vi "UI LED.vi"(8 "error in":errorcluster) -> (0 "error out":errorcluster)   [LabVIEW 2019, in "LED.lvlib"]
uses:
  LED.lvlib
  User Event/Controls/UE Abort Action.ctl
  SubVI/Image Para.ctl
  Camera/Andor/SubVI/seletion.ctl
  <vilib>/Utility/miscctls.llb/LVPointTypeDef.ctl
  SubVI/ADC Channel.ctl
  <vilib>/Utility/error.llb/Error Cluster From Error Code.vi
  <vilib>/ErrorRing/Error Ring.xnode
  Queues/Queues.lvlib
  Camera/Andor/Andor.lvlib
panel:
  in  "LED Control":T1={"LED"=enum."No Selection", "Power (%)"={"BrLED"=15, "Blue"=15, "Green"=15, "Red"=15, "UV"=15}} {"Power (%)"."UV" min=15 max=100; "Power (%)"."Red" min=15 max=100; "Power (%)"."Green" min=15 max=100; "Power (%)"."Blue" min=15 max=100; "Power (%)"."BrLED" min=15 max=100}
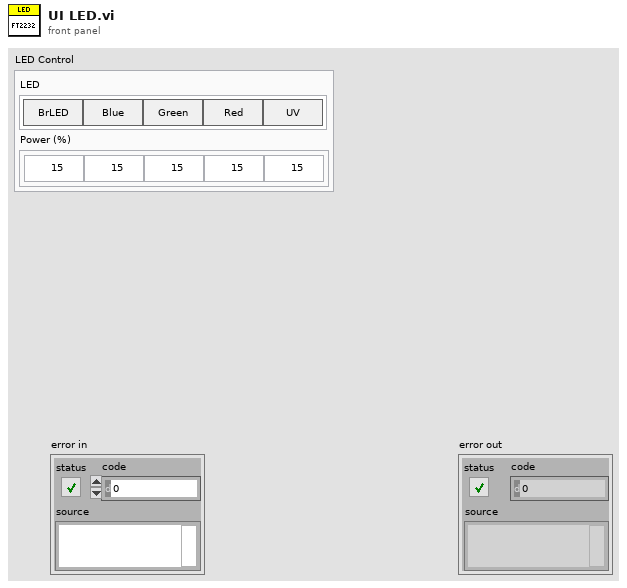
[diagram p1: front panel]
types:
  T1 = cluster{"LED":enum32{"No Selection", "BrLED", "Blue", "Green", "Red", "UV"}, "Power (%)":cluster{"BrLED":u8, "Blue":u8, "Green":u8, "Red":u8, "UV":u8}}
  T2 = cluster{"Initialize Sucess?":bool, "LED Control":cluster{"LED color":enum32{"BrLED", "Blue", "Green", "Red", "UV"}, "LED Power":u8}}
  T3 = typedef "UE Abort Action.ctl" = enum16{"Create", "Get", "Destroy"}
  T4 = typedef "LED.lvlib/Image Para.ctl" = cluster{"Marker":T5, "Power(Amp)":u8, "set shutter(s)":dbl, "Cube":enum16{"1", "2", "3", "4", "5", "6", "7", "8"}}
  T5 = typedef "Andor.lvlib/seletion.ctl" = enum16{"None", "Red", "Green", "Blue", "UV", "Green Laser", "Blue-Red", "UV-Red", "BF", "UV-IR"}
  T6 = cluster{"LED color":enum32{"BrLED", "Blue", "Green", "Red", "UV"}, "LED Power":u8}
  T7 = enum32{"No Selection", "BrLED", "Blue", "Green", "Red", "UV"}
  T8 = typedef "LVPointTypeDef.ctl" = cluster{"Horizontal":i16, "Vertical":i16}
  T9 = enum16{"LED Initial", "LED On", "LED Off", "LED Change", "LED Close", "ADC Read"}
  T10 = cluster{"return":i32, "numDev":u32, "ftHandleFluChA":u32, "ftHandleFluChB":u32, "ftHandleBriChA":u32, "ftHandleBriChB":u32, "ftHandelADCChA":u32, "ftHandleADCChB":u32}
  T11 = typedef "LED.lvlib/SEQ Data.ctl" = cluster{"Initialize Sucess?":bool, "BL2 Regulator":dbl, "BL1 Regulator":dbl, "Blood Sensor 1":dbl, "Blood Sensor 2":dbl, "Air Pressure Sensor":dbl, "Force Snesor 1":u32, "Force Snesor 2":u32, "VI Refnum":refnum<vi>}
  T12 = typedef "Rendezvous RefNum" = refnum<k1>
  T13 = typedef "LED.lvlib/ADC Channel.ctl" = enum16{"BL2 Regulator", "BL1 Regulator", "Blood Sensor 1", "Blood Sensor 2", "Air Pressure Sensor", "Force Sensor 1", "Force Snesor 2"}
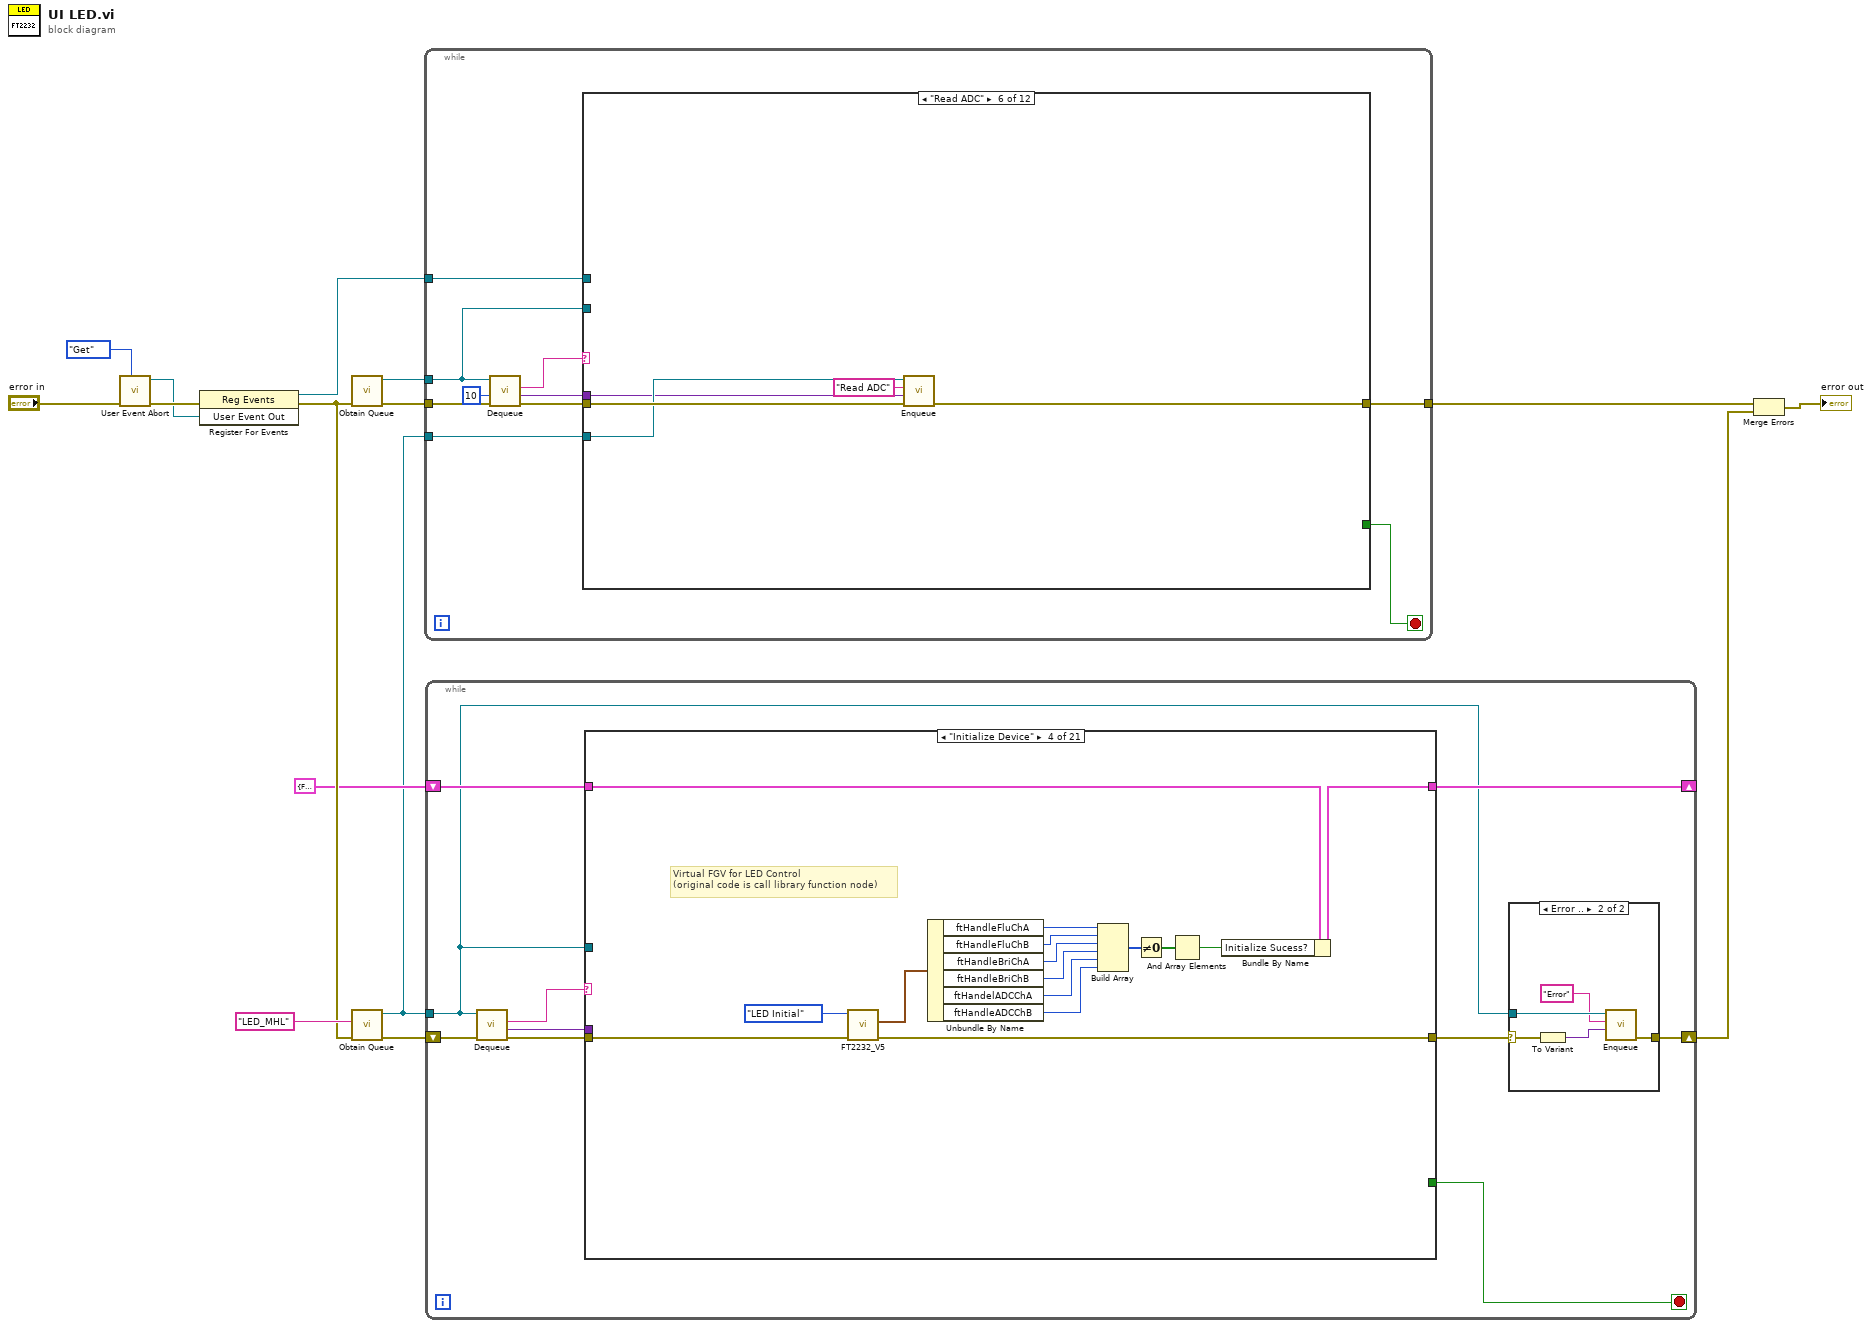
[diagram p0: block diagram]
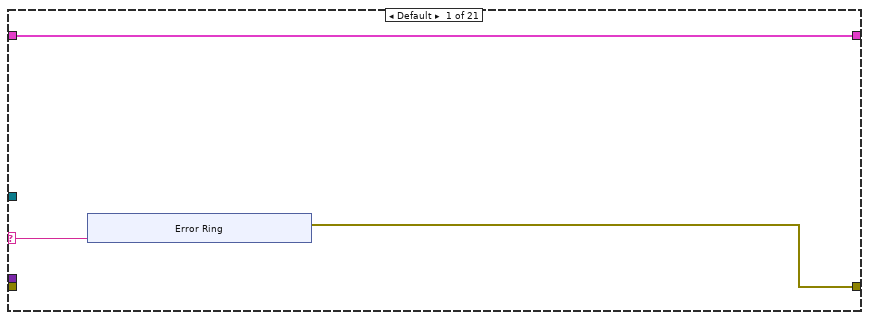
[diagram p2: hidden frame]
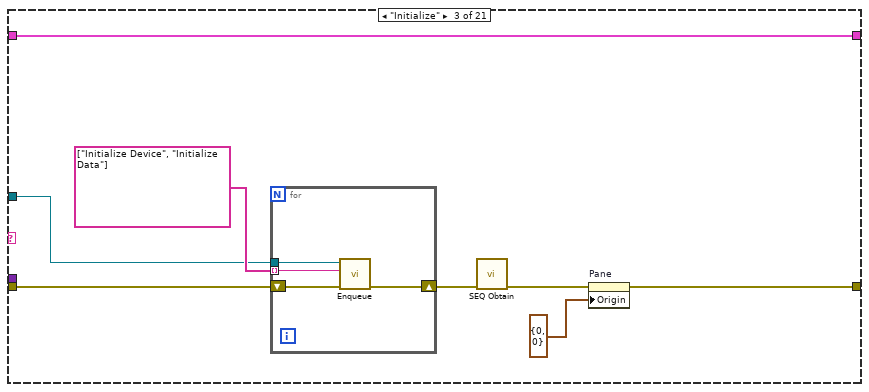
[diagram p4: hidden frame]
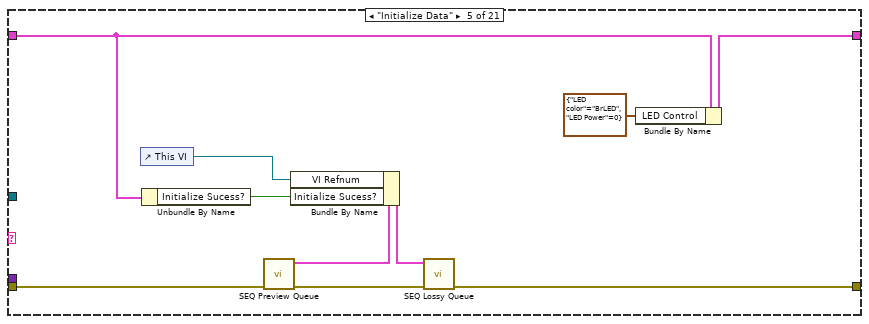
[diagram p5: hidden frame]
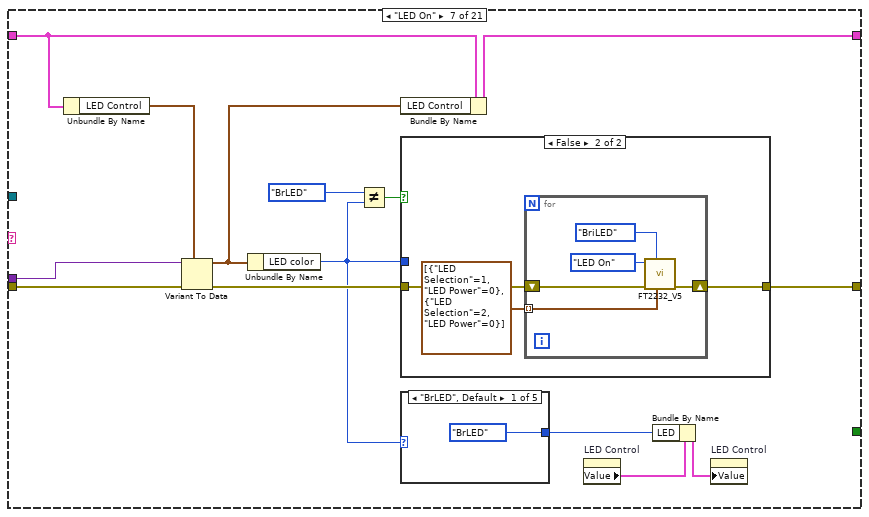
[diagram p7: hidden frame]
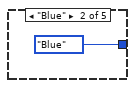
[diagram p8: hidden frame]
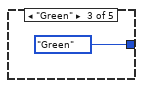
[diagram p9: hidden frame]
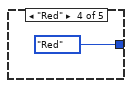
[diagram p10: hidden frame]
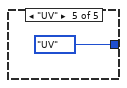
[diagram p11: hidden frame]
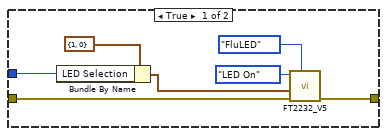
[diagram p12: hidden frame]
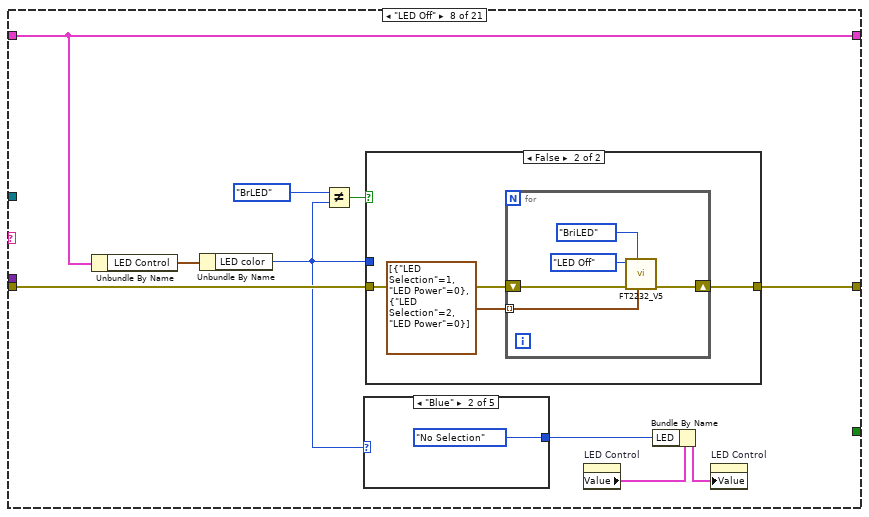
[diagram p13: hidden frame]
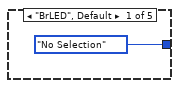
[diagram p14: hidden frame]
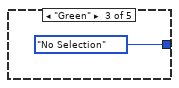
[diagram p15: hidden frame]
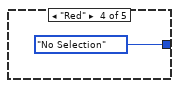
[diagram p16: hidden frame]
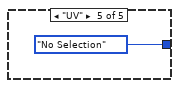
[diagram p17: hidden frame]
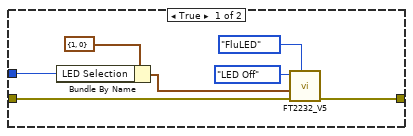
[diagram p18: hidden frame]
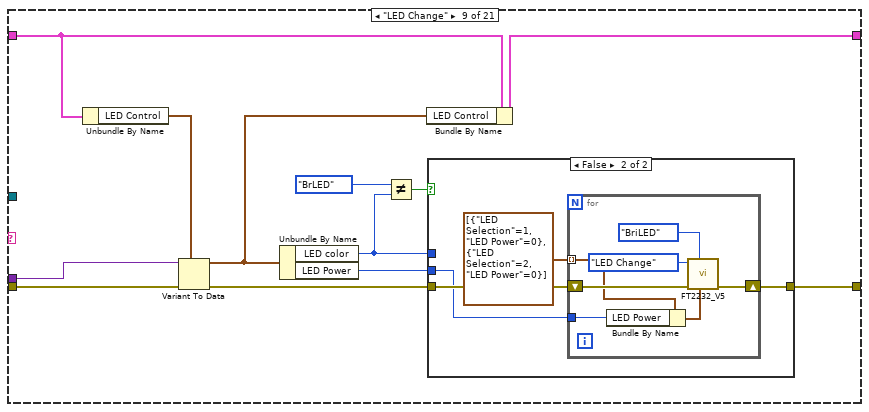
[diagram p19: hidden frame]
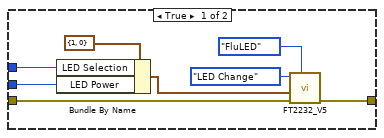
[diagram p20: hidden frame]
diagram:
  n1 = call "User Event Abort.vi"("Action"=UE_Abort_Action."Get", "Error In"="error in") -> ("Error Out"=w13:errorcluster, "User Event Out"=w12:refnum<user-event>)  [unwired: 8 in]
  n2 = register-events(error in=w13, w12) -> (reference out=w11:refnum<event-registration>, error out=w6:errorcluster)  [unwired: 1 in]
  n3 = call "Obtain Queue.vi"("Error In"=w6) -> ("Error Out"=w10:errorcluster, "Queue out"=w9:refnum<queue>)  [unwired: 9 in]
  n4 = call "Obtain Queue.vi"("Error In"=w6, "Queue Name"="LED_MHL") -> ("Error Out"=w7:errorcluster, "queue out"=w1:refnum<queue>)  [unwired: 8 in]
  n5 = while {
    tunnel: w10 -> [w25]
    tunnel: w9 -> [w20]
    tunnel: [w19] -> w5
    tunnel: w11 -> [w18]
    tunnel: w1 -> [w16]
    stop <- w17 stop-if-true
    n6 = call "Dequeue.vi"("Error In"=w25, "timeout in ms (-1)"=10, "Queue in"=w20) -> ("Error Out"=w24:errorcluster, "Data"=w22:variant, "State"=w23:string)  [unwired: 5 in, 1 out]
    n7 = case shown="\"Read ADC\"" w23 {
      selector: w23 -> [w26 _ _ _ _ _ _ _ _ _ _ _]
      tunnel: w24 -> [w29 w33 w52 w71 w77 w89 w93 w97 w100 w104 w108 w116]
      tunnel: w22 -> [_ _ w50 w69 _ w87 _ _ _ _ _ _]
      tunnel: w20 -> [_ _ _ _ _ _ _ _ _ _ _ _]
      tunnel: [w29 w32 w47 w66 w80 w86 w92 w96 w98 w103 w107 w115] -> w19
      tunnel: w18 -> [_ _ _ _ _ _ _ _ _ _ _ w114]
      tunnel: [_ _ _ _ _ _ _ _ _ _ TRUE _] -> w17
      tunnel: w16 -> [_ w31 w46 w65 w79 w88 w91 w95 w99 w102 w106 _]
      frame "Typo", Default {
        n8 = Concatenate Strings("Typo: " ("string"), w26) -> (w28:string)
        n9 = One Button Dialog(message=w28) -> ()  [unwired: 1 in, 1 out]
      }
      frame "Initialize" {
        n10 = for {
          tunnel: w31 -> [w35]
          shift-right: [w36] -> w32
          shift-left: w33 -> [w37]
          tunnel: string[] ["Initialize"] -> [w34] mode=indexing
          n11 = call "Enqueue.vi"("Error In"=w37, "State"=w34, "Queue in"=w35) -> ("Error Out"=w36:errorcluster)  [unwired: 7 in, 1 out]
        }
      }
      frame "LED On" {
        w44 = variant ("element")
        n12 = Variant To Data(error in=w52, type=T4 {"Marker"=enum."None", "Power(Amp)"=0, "set shutter(s)"=0.001, "Cube"=enum."2"} ("Color&Power control"), Variant=w50) -> (data=w48:T4, error out=w49:errorcluster)
        n13 = call "Image Para Extract.vi"("error in"=w49, "Image Para"=w48) -> ("error out"=w41:errorcluster, "LED Control out"=w39:T6)  [unwired: 6 in, 2 out]
        n14 = call "Power Convert.vi"("error in"=w41, "LED Control in"=w39) -> ("error out"=w40:errorcluster, "LED Control out"=w38:T6)  [unwired: 8 in]
        n15 = To Variant(anything=w38) -> (Variant=w45:variant)
        n16 = Build Array(w44, w44, w45, w45) -> (w43:variant[])
        n17 = for {
          tunnel: w46 -> [w55]
          shift-right: [w56] -> w47
          shift-left: w40 -> [w57]
          tunnel: w43 -> [w54] mode=indexing
          tunnel: string[] ["LED Zero", "LED Off", "LED Change", "LED On"] -> [w53] mode=indexing
          n18 = call "Enqueue.vi"("Error In"=w57, "Data"=w54, "State"=w53, "Queue in"=w55) -> ("Error Out"=w56:errorcluster)  [unwired: 6 in, 1 out]
        }
      }
      frame "LED Change" {
        n19 = Variant To Data(error in=w71, type=T4 {"Marker"=enum."None", "Power(Amp)"=0, "set shutter(s)"=0.001, "Cube"=enum."2"} ("Color&Power control"), Variant=w69) -> (data=w67:T4, error out=w68:errorcluster)
        n20 = call "Image Para Extract.vi"("error in"=w68, "Image Para"=w67) -> ("error out"=w61:errorcluster, "LED Control out"=w59:T6)  [unwired: 6 in, 2 out]
        n21 = call "Power Convert.vi"("error in"=w61, "LED Control in"=w59) -> ("error out"=w60:errorcluster, "LED Control out"=w58:T6)  [unwired: 8 in]
        n22 = To Variant(anything=w58) -> (Variant=w62:variant)
        n23 = Build Array(w62) -> (w64:variant[])
        n24 = for {
          tunnel: w65 -> [w74]
          shift-right: [w75] -> w66
          shift-left: w60 -> [w76]
          tunnel: w64 -> [w73] mode=indexing
          tunnel: string[] ["LED Change"] -> [w72] mode=indexing
          n25 = call "Enqueue.vi"("Error In"=w76, "Data"=w73, "State"=w72, "Queue in"=w74) -> ("Error Out"=w75:errorcluster)  [unwired: 6 in, 1 out]
        }
      }
      frame "LED Off" {
        n26 = for {
          tunnel: w79 -> [w82]
          shift-right: [w83] -> w80
          shift-left: w77 -> [w84]
          tunnel: string[] ["LED Zero", "LED Off"] -> [w81] mode=indexing
          n27 = call "Enqueue.vi"("Error In"=w84, "State"=w81, "Queue in"=w82) -> ("Error Out"=w83:errorcluster)  [unwired: 7 in, 1 out]
        }
      }
      frame "Read ADC" {
        n28 = call "Enqueue.vi"("Error In"=w89, "Data"=w87, "State"="Read ADC", "Queue in"=w88) -> ("Error Out"=w86:errorcluster)  [unwired: 6 in, 1 out]
      }
      frame "Read BL2 Regulator" {
        n29 = call "Enqueue.vi"("Error In"=w93, "State"="Read BL2 Regulator", "Queue in"=w91) -> ("Error Out"=w92:errorcluster)  [unwired: 7 in, 1 out]
      }
      frame "Read Force Sensor" {
        n30 = call "Enqueue.vi"("Error In"=w97, "State"="Read Force Sensor 1", "Queue in"=w95) -> ("Error Out"=w96:errorcluster)  [unwired: 7 in, 1 out]
      }
      frame "Stop Read" {
        n31 = Flush Queue(queue=w99, error in (no error)=w100) -> (error out=w98:errorcluster)  [unwired: 2 out]
      }
      frame "Rendezvous Acquire" {
        n32 = call "Enqueue.vi"("Error In"=w104, "State"="Rendezvous Acquire", "Queue in"=w102) -> ("Error Out"=w103:errorcluster)  [unwired: 7 in, 1 out]
      }
      frame "Close" {
        n33 = for {
          tunnel: w106 -> [w111]
          shift-right: [w112] -> w107
          shift-left: w108 -> [w113]
          tunnel: string[] ["LED Zero", "LED Off", "Close"] -> [w110] mode=indexing
          n34 = call "Enqueue.vi"("Error In"=w113, "State"=w110, "Queue in"=w111) -> ("Error Out"=w112:errorcluster)  [unwired: 7 in, 1 out]
        }
      }
      frame "Idle" {
        n35 = event shown="[1] \"LED Control.LED\": Value Change" {
          selector: w114 -> [_ _ w163]
          dyn-events: _ -> [_ _ _]
          timeout: 10 -> [_ _ _]
          tunnel: w116 -> [w118 w121 w161]
          tunnel: [w118 w120 w162] -> w115
          event Timeout {
            n36 = event-data() -> ()  [unwired: 1 in, 3 out]
          }
          event "LED Control.LED": Value Change {
            n37 = event-data() -> ("NewVal"=w122:T7)  [unwired: 1 in, 5 out]
            n38 = case shown="\"No Selection\", Default" w122 {
              tunnel: w121 -> [w124 w131 w134 w141 w148 w155]
              tunnel: [w123 w130 w133 w140 w147 w154] -> w120
              tunnel: "LED Control" -> [_ w129 w132 w139 w146 w153]
              frame "No Selection", Default {
                n39 = call "LED Off.vi"("Error In"=w124) -> ("Error Out"=w123:errorcluster)  [unwired: 10 in]
              }
              frame "BrLED" {
                n40 = Unbundle By Name(w129) -> ("Power (%).BrLED"=w127:u8)
                n41 = Bundle By Name(cluster=T4 {"Marker"=enum."None", "Power(Amp)"=15, "set shutter(s)"=0.001, "Cube"=enum."1"} ("Image Para"), "Marker"=seletion."BF", "Power(Amp)"=w127) -> (w125:T4)
                n42 = call "LED On.vi"("Error In"=w131, "Image Para"=w125) -> ("Error Out"=w130:errorcluster)  [unwired: 9 in]
              }
              frame "Blue" {
                n43 = Unbundle By Name(w132) -> ("Power (%).Blue"=w137:u8)
                n44 = Bundle By Name(cluster=T4 {"Marker"=enum."None", "Power(Amp)"=15, "set shutter(s)"=0.001, "Cube"=enum."1"} ("Image Para"), "Marker"=seletion."Blue", "Power(Amp)"=w137) -> (w135:T4)
                n45 = call "LED On.vi"("Error In"=w134, "Image Para"=w135) -> ("Error Out"=w133:errorcluster)  [unwired: 9 in]
              }
              frame "Green" {
                n46 = Unbundle By Name(w139) -> ("Power (%).Green"=w144:u8)
                n47 = Bundle By Name(cluster=T4 {"Marker"=enum."None", "Power(Amp)"=15, "set shutter(s)"=0.001, "Cube"=enum."1"} ("Image Para"), "Marker"=seletion."Green", "Power(Amp)"=w144) -> (w142:T4)
                n48 = call "LED On.vi"("Error In"=w141, "Image Para"=w142) -> ("Error Out"=w140:errorcluster)  [unwired: 9 in]
              }
              frame "Red" {
                n49 = Unbundle By Name(w146) -> ("Power (%).Red"=w151:u8)
                n50 = Bundle By Name(cluster=T4 {"Marker"=enum."None", "Power(Amp)"=15, "set shutter(s)"=0.001, "Cube"=enum."1"} ("Image Para"), "Marker"=seletion."Red", "Power(Amp)"=w151) -> (w149:T4)
                n51 = call "LED On.vi"("Error In"=w148, "Image Para"=w149) -> ("Error Out"=w147:errorcluster)  [unwired: 9 in]
              }
              frame "UV" {
                n52 = Unbundle By Name(w153) -> ("Power (%).UV"=w158:u8)
                n53 = Bundle By Name(cluster=T4 {"Marker"=enum."None", "Power(Amp)"=15, "set shutter(s)"=0.001, "Cube"=enum."1"} ("Image Para"), "Marker"=seletion."UV", "Power(Amp)"=w158) -> (w156:T4)
                n54 = call "LED On.vi"("Error In"=w155, "Image Para"=w156) -> ("Error Out"=w154:errorcluster)  [unwired: 9 in]
              }
            }
          }
          event User Event {
            n55 = event-data() -> ()  [unwired: 1 in, 4 out]
            n56 = call "Close.vi"("Error In"=w161) -> ("Error Out"=w160:errorcluster)  [unwired: 10 in]
            n57 = Unregister For Events(event registration refnum=w163, error in=w160) -> (error out=w162:errorcluster)
          }
        }
      }
    }
  }
  n58 = while {
    tunnel: w1 -> [w165]
    shift-right: [w168] -> _
    shift-left: T2 {"Initialize Sucess?"=FALSE, "LED Control"={"LED color"=enum."BrLED", "LED Power"=0}} -> [w169]
    shift-right: [w167] -> w3
    shift-left: w7 -> [w173]
    stop <- w164 stop-if-true
    n59 = call "Dequeue.vi"("Error In"=w173, "Queue in"=w165) -> ("Error Out"=w170:errorcluster, "Data"=w171:variant, "State"=w172:string)  [unwired: 6 in, 1 out]
    n60 = case shown="\"Initialize Device\"" w172 {
      selector: w172 -> [w175 _ _ _ _ _ _ _ _ _ _ _ _ _ _ _ _ _ _ _ _]
      tunnel: w165 -> [_ _ w191 _ _ _ _ _ _ _ _ _ w406 w420 w436 _ _ _ w460 _ w471]
      tunnel: w171 -> [_ _ _ _ _ _ w233 _ w295 _ _ w375 _ _ _ _ w452 _ _ _ _]
      tunnel: w170 -> [_ w184 w192 w202 w219 w224 w235 w266 w297 w324 w355 w376 w408 w422 w438 w449 w453 w457 w461 w469 w474]
      tunnel: w169 -> [w176 w185 w189 w200 w217 w223 w232 w264 w294 w323 w356 w378 w418 w432 w447 w448 w450 w456 w458 w467 w476]
      tunnel: [w176 w185 w189 w199 w215 w223 w230 w264 w292 w323 w356 w378 w418 w432 w447 w448 w450 w456 w458 w467 w476] -> w168
      tunnel: [w174 w184 w186 w201 w218 w224 w236 w265 w298 w325 w347 w368 w413 w427 w442 w449 errorcluster {"status"=FALSE, "code"=0, "source"=""} ("Error Out") w457 w459 w468 w472] -> w166
      tunnel: [_ _ _ _ _ _ _ _ _ _ _ _ _ _ _ _ _ _ _ _ TRUE] -> w164
      frame Default {
        n61 = xnode "Error Ring"("parameter 0"=w175) -> ("error out"=w174:errorcluster)
      }
      frame "------Initialize------" {
      }
      frame "Initialize" {
        n62 = for {
          tunnel: w191 -> [w195]
          shift-right: [w196] -> w190
          shift-left: w192 -> [w197]
          tunnel: string[] ["Initialize Device", "Initialize Data"] -> [w194] mode=indexing
          n63 = call "Enqueue.vi"("Error In"=w197, "State"=w194, "Queue in"=w195) -> ("Error Out"=w196:errorcluster)  [unwired: 7 in, 1 out]
        }
        n64 = call "SEQ Obtain.vi"("error in"=w190) -> ("error out"=w188:errorcluster)  [unwired: 9 in, 1 out]
        n65 = property on="Pane" class="Pane"(error in=w188, "Origin"=T8 {"Horizontal"=0, "Vertical"=0}) -> (error out=w186:errorcluster)  [unwired: 1 in, 1 out]
      }
      frame "Initialize Device" {
        # "Virtual FGV for LED Control\n(original code is call library function node)"
        n66 = call "FT2232_V5.vi"("error in"=w202, "LED event"=T9."LED Initial") -> ("error out"=w201:errorcluster, "Initialize"=w204:T10)  [unwired: 6 in, 2 out]
        n67 = Unbundle By Name(w204) -> ("ftHandleFluChA"=w205:u32, "ftHandleFluChB"=w206:u32, "ftHandleBriChA"=w207:u32, "ftHandleBriChB"=w208:u32, "ftHandelADCChA"=w209:u32, "ftHandleADCChB"=w210:u32)
        n68 = Build Array(w205, w206, w207, w208, w209, w210) -> (w211:u32[])
        n69 = Not Equal To 0?(x=w211) -> (x != 0?=w212:bool[])
        n70 = And Array Elements(Boolean array=w212) -> (logical AND=w198:bool)
        n71 = Bundle By Name(cluster=w200, "Initialize Sucess?"=w198) -> (w199:T2)
      }
      frame "Initialize Data" {
        n72 = control-ref of="This VI"() -> (w213:refnum<vi>)
        n73 = Unbundle By Name(w217) -> ("Initialize Sucess?"=w216:bool)
        n74 = call "SEQ Preview Queue.vi"("error in"=w219) -> ("error out"=w220:errorcluster, "SEQ Data"=w221:T11)  [unwired: 9 in]
        n75 = Bundle By Name(cluster=w221, "VI Refnum"=w213, "Initialize Sucess?"=w216) -> (w222:T11)
        n76 = call "SEQ Lossy Queue.vi"("error in"=w220, "SEQ Data"=w222) -> ("error out"=w218:errorcluster)  [unwired: 9 in]
        n77 = Bundle By Name(cluster=w217, "LED Control"=T6 {"LED color"=enum."BrLED", "LED Power"=0}) -> (w215:T2)
      }
      frame "------Functions------" {
      }
      frame "LED On" {
        n78 = Unbundle By Name(w232) -> ("LED Control"=w231:T6)
        n79 = Variant To Data(error in=w235, type=w231, Variant=w233) -> (data=w229:T6, error out=w234:errorcluster)
        n80 = Unbundle By Name(w229) -> ("LED color"=w226:enum32{"BrLED", "Blue", "Green", "Red", "UV"})
        n81 = Not Equal?(x=enum32{"BrLED", "Blue", "Green", "Red", "UV"}."BrLED", y=w226) -> (x != y?=w238:bool)
        n82 = Bundle By Name(cluster=w232, "LED Control"=w229) -> (w230:T2)
        n83 = case shown="False" w238 {
          tunnel: w234 -> [w250 w253]
          tunnel: [w244 w251] -> w236
          tunnel: w226 -> [w246 _]
          frame True {
            n84 = Bundle By Name(cluster=cluster{"LED Selection":u16, "LED Power":u8} {"LED Selection"=1, "LED Power"=0} ("FulLED set"), "LED Selection"=w246) -> (w245:cluster{"LED Selection":u16, "LED Power":u8})
            n85 = call "FT2232_V5.vi"("LED selection"=enum16{"FluLED", "BriLED", "ADCDAC"}."FluLED", "error in"=w250, "FulLED set"=w245, "LED event"=T9."LED On") -> ("error out"=w244:errorcluster)  [unwired: 4 in, 3 out]
          }
          frame False {
            n86 = for {
              shift-right: [w254] -> w251
              shift-left: w253 -> [w258]
              tunnel: cluster{"LED Selection":u16, "LED Power":u8}[] [{"LED Selection"=1, "LED Power"=0}, {"LED Selection"=2, "LED Power"=0}] -> [w255] mode=indexing
              n87 = call "FT2232_V5.vi"("BriLED set"=w255, "LED selection"=enum16{"FluLED", "BriLED", "ADCDAC"}."BriLED", "error in"=w258, "LED event"=T9."LED On") -> ("error out"=w254:errorcluster)  [unwired: 4 in, 3 out]
            }
          }
        }
        n88 = case shown="\"BrLED\", Default" w226 {
          tunnel: [T7."BrLED" ("LED") T7."Blue" ("LED") T7."Green" ("LED") T7."Red" ("LED") T7."UV" ("LED")] -> w225
          frame "BrLED", Default {
          }
          frame "Blue" {
          }
          frame "Green" {
          }
          frame "Red" {
          }
          frame "UV" {
          }
        }
        n89 = property on="LED Control" class="Clust (strict)"() -> ("Value"=w228:T1)  [unwired: 2 in, 2 out]
        n90 = Bundle By Name(cluster=w228, "LED"=w225) -> (w227:T1)
        n91 = property on="LED Control" class="Clust (strict)"("Value"=w227) -> ()  [unwired: 2 in, 2 out]
      }
      frame "LED Off" {
        n92 = Unbundle By Name(w264) -> ("LED Control"=w263:T6)
        n93 = Unbundle By Name(w263) -> ("LED color"=w259:enum32{"BrLED", "Blue", "Green", "Red", "UV"})
        n94 = Not Equal?(x=enum32{"BrLED", "Blue", "Green", "Red", "UV"}."BrLED", y=w259) -> (x != y?=w268:bool)
        n95 = case shown="\"Blue\"" w259 {
          tunnel: [T7."No Selection" ("LED") T7."No Selection" ("LED") T7."No Selection" ("LED") T7."No Selection" ("LED") T7."No Selection" ("LED")] -> w260
          frame "BrLED", Default {
          }
          frame "Blue" {
          }
          frame "Green" {
          }
          frame "Red" {
          }
          frame "UV" {
          }
        }
        n96 = case shown="False" w268 {
          tunnel: w266 -> [w280 w283]
          tunnel: [w274 w282] -> w265
          tunnel: w259 -> [w276 _]
          frame True {
            n97 = Bundle By Name(cluster=cluster{"LED Selection":u16, "LED Power":u8} {"LED Selection"=1, "LED Power"=0} ("FulLED set"), "LED Selection"=w276) -> (w275:cluster{"LED Selection":u16, "LED Power":u8})
            n98 = call "FT2232_V5.vi"("LED selection"=enum16{"FluLED", "BriLED", "ADCDAC"}."FluLED", "error in"=w280, "FulLED set"=w275, "LED event"=T9."LED Off") -> ("error out"=w274:errorcluster)  [unwired: 4 in, 3 out]
          }
          frame False {
            n99 = for {
              shift-right: [w284] -> w282
              shift-left: w283 -> [w288]
              tunnel: cluster{"LED Selection":u16, "LED Power":u8}[] [{"LED Selection"=1, "LED Power"=0}, {"LED Selection"=2, "LED Power"=0}] -> [w285] mode=indexing
              n100 = call "FT2232_V5.vi"("BriLED set"=w285, "LED selection"=enum16{"FluLED", "BriLED", "ADCDAC"}."BriLED", "error in"=w288, "LED event"=T9."LED Off") -> ("error out"=w284:errorcluster)  [unwired: 4 in, 3 out]
            }
          }
        }
        n101 = property on="LED Control" class="Clust (strict)"() -> ("Value"=w262:T1)  [unwired: 2 in, 2 out]
        n102 = Bundle By Name(cluster=w262, "LED"=w260) -> (w261:T1)
        n103 = property on="LED Control" class="Clust (strict)"("Value"=w261) -> ()  [unwired: 2 in, 2 out]
      }
      frame "LED Change" {
        n104 = Unbundle By Name(w294) -> ("LED Control"=w293:T6)
        n105 = Variant To Data(error in=w297, type=w293, Variant=w295) -> (data=w291:T6, error out=w296:errorcluster)
        n106 = Unbundle By Name(w291) -> ("LED color"=w290:enum32{"BrLED", "Blue", "Green", "Red", "UV"}, "LED Power"=w289:u8)
        n107 = Not Equal?(x=enum32{"BrLED", "Blue", "Green", "Red", "UV"}."BrLED", y=w290) -> (x != y?=w300:bool)
        n108 = Bundle By Name(cluster=w294, "LED Control"=w291) -> (w292:T2)
        n109 = case shown="False" w300 {
          tunnel: w296 -> [w308 w312]
          tunnel: [w301 w311] -> w298
          tunnel: w290 -> [w304 _]
          tunnel: w289 -> [w302 w309]
          frame True {
            n110 = Bundle By Name(cluster=cluster{"LED Selection":u16, "LED Power":u8} {"LED Selection"=1, "LED Power"=0} ("FulLED set"), "LED Selection"=w304, "LED Power"=w302) -> (w303:cluster{"LED Selection":u16, "LED Power":u8})
            n111 = call "FT2232_V5.vi"("LED selection"=enum16{"FluLED", "BriLED", "ADCDAC"}."FluLED", "error in"=w308, "FulLED set"=w303, "LED event"=T9."LED Change") -> ("error out"=w301:errorcluster)  [unwired: 4 in, 3 out]
          }
          frame False {
            n112 = for {
              shift-right: [w313] -> w311
              shift-left: w312 -> [w319]
              tunnel: cluster{"LED Selection":u16, "LED Power":u8}[] [{"LED Selection"=1, "LED Power"=0}, {"LED Selection"=2, "LED Power"=0}] -> [w316] mode=indexing
              tunnel: w309 -> [w314]
              n113 = Bundle By Name(cluster=w316, "LED Power"=w314) -> (w315:cluster{"LED Selection":u16, "LED Power":u8})
              n114 = call "FT2232_V5.vi"("BriLED set"=w315, "LED selection"=enum16{"FluLED", "BriLED", "ADCDAC"}."BriLED", "error in"=w319, "LED event"=T9."LED Change") -> ("error out"=w313:errorcluster)  [unwired: 4 in, 3 out]
            }
          }
        }
      }
      frame "LED Zero" {
        n115 = Unbundle By Name(w323) -> ("LED Control"=w322:T6)
        n116 = Unbundle By Name(w322) -> ("LED color"=w321:enum32{"BrLED", "Blue", "Green", "Red", "UV"})
        n117 = Not Equal?(x=enum32{"BrLED", "Blue", "Green", "Red", "UV"}."BrLED", y=w321) -> (x != y?=w327:bool)
        n118 = case shown="True" w327 {
          tunnel: w324 -> [w335 w339]
          tunnel: [w328 w338] -> w325
          tunnel: w321 -> [w331 _]
          tunnel: u8 0 ("LED Power") -> [w329 w336]
          frame True {
            n119 = Bundle By Name(cluster=cluster{"LED Selection":u16, "LED Power":u8} {"LED Selection"=1, "LED Power"=0} ("FulLED set"), "LED Selection"=w331, "LED Power"=w329) -> (w330:cluster{"LED Selection":u16, "LED Power":u8})
            n120 = call "FT2232_V5.vi"("LED selection"=enum16{"FluLED", "BriLED", "ADCDAC"}."FluLED", "error in"=w335, "FulLED set"=w330, "LED event"=T9."LED Change") -> ("error out"=w328:errorcluster)  [unwired: 4 in, 3 out]
          }
          frame False {
            n121 = for {
              shift-right: [w340] -> w338
              shift-left: w339 -> [w346]
              tunnel: cluster{"LED Selection":u16, "LED Power":u8}[] [{"LED Selection"=1, "LED Power"=0}, {"LED Selection"=2, "LED Power"=0}] -> [w343] mode=indexing
              tunnel: w336 -> [w341]
              n122 = Bundle By Name(cluster=w343, "LED Power"=w341) -> (w342:cluster{"LED Selection":u16, "LED Power":u8})
              n123 = call "FT2232_V5.vi"("BriLED set"=w342, "LED selection"=enum16{"FluLED", "BriLED", "ADCDAC"}."BriLED", "error in"=w346, "LED event"=T9."LED Change") -> ("error out"=w340:errorcluster)  [unwired: 4 in, 3 out]
            }
          }
        }
      }
      frame "Rendezvous Acquire" {
        n124 = call <vilib>:"Create Rendezvous.vi"("error in (no error)"=w355, "size (2)"=4, "name (unnamed)"="Acquire") -> ("error out"=w354:errorcluster, "rendezvous"=w353:T12)  [unwired: 2 in, 1 out]
        n125 = call <vilib>:"Wait at Rendezvous.vi"("error in (no error)"=w354, "ms timeout (-1)"=10000, "rendezvous"=w353) -> ("error out"=w349:errorcluster, "timed out"=w348:bool)  [unwired: 2 in, 1 out]
        n126 = case shown="True" w348 {
          tunnel: w349 -> [w357 _]
          tunnel: [w357 w358] -> w347
          frame False {
          }
          frame True {
            n127 = xnode "Error Ring"() -> ("error out"=w358:errorcluster)
          }
        }
      }
      frame "Read ADC" {
        w374 = ADC_Channel."BL2 Regulator"  # ADC Channel
        n128 = Variant To Data(error in=w376, type=w374, Variant=w375) -> (data=w365:T13, error out=w372:errorcluster)
        n129 = To Unsigned Word Integer(number=w365) -> (unsigned 16bit integer=w373:u16)
        n130 = Wait (ms)(milliseconds to wait=u32 100) -> ()  [unwired: 1 out]
        n131 = call "FT2232_V5.vi"("error in"=w372, "ADC_Channel"=w373, "LED event"=T9."ADC Read") -> ("error out"=w370:errorcluster, "ADC_Data"=w364:u32)  [unwired: 5 in, 2 out]
        n132 = call "SEQ Preview Queue.vi"("error in"=w370) -> ("error out"=w369:errorcluster, "SEQ Data"=w367:T11)  [unwired: 9 in]
        n133 = case shown="\"BL2 Regulator\", Default" w365 {
          tunnel: w367 -> [w381 w386 w389 w393 w397 w400 w403]
          tunnel: [w382 w385 w390 w394 w398 w401 w404] -> w366
          tunnel: w364 -> [w380 w384 w388 w392 w396 w399 w402]
          frame "BL2 Regulator", Default {
            n134 = call "ADC Converter.vi"("ADC in"=w380) -> ("ADC out"=w379:dbl)  [unwired: 9 in, 1 out]
            n135 = Bundle By Name(cluster=w381, "BL2 Regulator"=w379) -> (w382:T11)
          }
          frame "BL1 Regulator" {
            n136 = call "ADC Converter.vi"("ADC in"=w384) -> ("ADC out"=w383:dbl)  [unwired: 9 in, 1 out]
            n137 = Bundle By Name(cluster=w386, "BL1 Regulator"=w383) -> (w385:T11)
          }
          frame "Blood Sensor 1" {
            n138 = call "ADC Converter.vi"("ADC in"=w388) -> ("ADC out"=w387:dbl)  [unwired: 9 in, 1 out]
            n139 = Bundle By Name(cluster=w389, "Blood Sensor 1"=w387) -> (w390:T11)
          }
          frame "Blood Sensor 2" {
            n140 = call "ADC Converter.vi"("ADC in"=w392) -> ("ADC out"=w391:dbl)  [unwired: 9 in, 1 out]
            n141 = Bundle By Name(cluster=w393, "Blood Sensor 2"=w391) -> (w394:T11)
          }
          frame "Air Pressure Sensor" {
            n142 = call "ADC Converter.vi"("ADC in"=w396) -> ("ADC out"=w395:dbl)  [unwired: 9 in, 1 out]
            n143 = Bundle By Name(cluster=w397, "Air Pressure Sensor"=w395) -> (w398:T11)
          }
          frame "Force Sensor 1" {
            n144 = Bundle By Name(cluster=w400, "Force Snesor 1"=w399) -> (w401:T11)
          }
          frame "Force Snesor 2" {
            n145 = Bundle By Name(cluster=w403, "Force Snesor 2"=w402) -> (w404:T11)
          }
        }
        n146 = call "SEQ Lossy Queue.vi"("error in"=w369, "SEQ Data"=w366) -> ("error out"=w368:errorcluster)  [unwired: 9 in]
      }
      frame "Read Force Sensor 1" {
        n147 = call "Enqueue.vi"("Error In"=w408, "State"="Read Force Sensor 2", "Queue in"=w406) -> ("Error Out"=w407:errorcluster)  [unwired: 7 in, 1 out]
        n148 = call "FT2232_V5.vi"("error in"=w407, "ADC_Channel"=u32 5, "LED event"=T9."ADC Read") -> ("error out"=w415:errorcluster, "ADC_Data"=w410:u32)  [unwired: 5 in, 2 out]
        n149 = Wait (ms)(milliseconds to wait=u32 200) -> ()  [unwired: 1 out]
        n150 = call "SEQ Preview Queue.vi"("error in"=w415) -> ("error out"=w414:errorcluster, "SEQ Data"=w412:T11)  [unwired: 9 in]
        n151 = Bundle By Name(cluster=w412, "Force Snesor 1"=w410) -> (w411:T11)
        n152 = call "SEQ Lossy Queue.vi"("error in"=w414, "SEQ Data"=w411) -> ("error out"=w413:errorcluster)  [unwired: 9 in]
      }
      frame "Read Force Sensor 2" {
        n153 = call "Enqueue.vi"("Error In"=w422, "State"="Read Force Sensor 1", "Queue in"=w420) -> ("Error Out"=w421:errorcluster)  [unwired: 7 in, 1 out]
        n154 = call "FT2232_V5.vi"("error in"=w421, "ADC_Channel"=u32 6, "LED event"=T9."ADC Read") -> ("error out"=w429:errorcluster, "ADC_Data"=w424:u32)  [unwired: 5 in, 2 out]
        n155 = Wait (ms)(milliseconds to wait=u32 200) -> ()  [unwired: 1 out]
        n156 = call "SEQ Preview Queue.vi"("error in"=w429) -> ("error out"=w428:errorcluster, "SEQ Data"=w426:T11)  [unwired: 9 in]
        n157 = Bundle By Name(cluster=w426, "Force Snesor 2"=w424) -> (w425:T11)
        n158 = call "SEQ Lossy Queue.vi"("error in"=w428, "SEQ Data"=w425) -> ("error out"=w427:errorcluster)  [unwired: 9 in]
      }
      frame "Read BL2 Regulator" {
        n159 = call "Enqueue.vi"("Error In"=w438, "State"="Read BL2 Regulator", "Queue in"=w436) -> ("Error Out"=w437:errorcluster)  [unwired: 7 in, 1 out]
        n160 = call "FT2232_V5.vi"("error in"=w437, "ADC_Channel"=u32 0, "LED event"=T9."ADC Read") -> ("error out"=w444:errorcluster, "ADC_Data"=w434:u32)  [unwired: 5 in, 2 out]
        n161 = Wait (ms)(milliseconds to wait=u32 200) -> ()  [unwired: 1 out]
        n162 = call "ADC Converter.vi"("ADC in"=w434) -> ("ADC out"=w433:dbl)  [unwired: 9 in, 1 out]
        n163 = call "SEQ Preview Queue.vi"("error in"=w444) -> ("error out"=w443:errorcluster, "SEQ Data"=w441:T11)  [unwired: 9 in]
        n164 = Bundle By Name(cluster=w441, "BL2 Regulator"=w433) -> (w440:T11)
        n165 = call "SEQ Lossy Queue.vi"("error in"=w443, "SEQ Data"=w440) -> ("error out"=w442:errorcluster)  [unwired: 9 in]
      }
      frame "------Error Handler------" {
      }
      frame "Error" {
        n166 = Variant To Data(error in=w453, type=errorcluster {"status"=FALSE, "code"=0, "source"=""} ("error constant"), Variant=w452) -> (data=w454:errorcluster)  [unwired: 1 out]
        n167 = call <vilib>:"Simple Error Handler.vi"("error in (no error)"=w454) -> ()  [unwired: 4 in, 5 out]
      }
      frame "------Close------" {
      }
      frame "Close" {
        n168 = for {
          tunnel: w460 -> [w464]
          shift-right: [w465] -> w459
          shift-left: w461 -> [w466]
          tunnel: string[] ["Close Device", "Release Queue"] -> [w463] mode=indexing
          n169 = call "Enqueue.vi"("Error In"=w466, "State"=w463, "Queue in"=w464) -> ("Error Out"=w465:errorcluster)  [unwired: 7 in, 1 out]
        }
      }
      frame "Close Device" {
        n170 = call "FT2232_V5.vi"("error in"=w469, "LED event"=T9."LED Close") -> ("error out"=w468:errorcluster)  [unwired: 6 in, 3 out]
      }
      frame "Release Queue" {
        n171 = Release Queue(queue=w471, error in (no error)=w474) -> (error out=w473:errorcluster)  [unwired: 1 in, 2 out]
        n172 = call "SEQ Release Queue.vi"("error in"=w473) -> ("error out"=w472:errorcluster)  [unwired: 10 in]
      }
    }
    n173 = case shown="Error .." w166 {
      selector: w166 -> [w477 w481]
      tunnel: [w477 w482] -> w167
      tunnel: w165 -> [_ w479]
      frame No Error {
      }
      frame Error {
        n174 = To Variant(anything=w481) -> (Variant=w480:variant)
        n175 = call "Enqueue.vi"("Data"=w480, "State"="Error", "Queue in"=w479) -> ("Error Out"=w482:errorcluster)  [unwired: 7 in, 1 out]
      }
    }
  }
  n176 = Merge Errors(w5, w3) -> (→"error out":errorcluster)
